vi "in loop button properties.vi"(0 "range settings":T1, 7 "range indicator refs":T2, 11 "error in (no error)":errorcluster) -> (15 "error out":errorcluster)   [LabVIEW 2014]
doc: "This subvi manages the boolean indicator properties inside the main temperature controller loop.\n\nPaul K Dixon\nPhysics 350\nPaul K Dixon"
uses:
  typedefs/status indicator.ctl
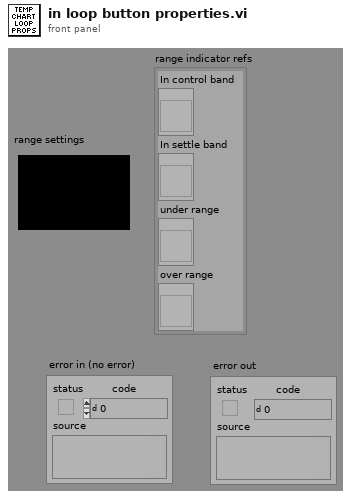
[diagram p1: front panel]
types:
  T1 = typedef "status indicator.ctl" = cluster{"In control band":bool, "In settle band":bool, "under range":bool, "over range":bool}
  T2 = cluster{"In control band":refnum<vi>, "In settle band":refnum<vi>, "under range":refnum<vi>, "over range":refnum<vi>}
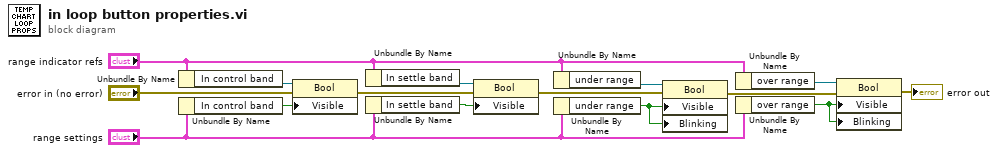
[diagram p0: block diagram]
diagram:
  n1 = Unbundle By Name("range indicator refs") -> ("In control band"=w15:refnum<vi>)
  n2 = Unbundle By Name("range settings") -> ("In control band"=w5:bool)
  n3 = property class="Bool"(reference=w15, error in="error in (no error)", "Visible"=w5) -> (error out=w12:errorcluster)  [unwired: 1 out]
  n4 = Unbundle By Name("range indicator refs") -> ("In settle band"=w13:refnum<vi>)
  n5 = Unbundle By Name("range settings") -> ("In settle band"=w3:bool)
  n6 = property class="Bool"(reference=w13, error in=w12, "Visible"=w3) -> (error out=w11:errorcluster)  [unwired: 1 out]
  n7 = Unbundle By Name("range indicator refs") -> ("under range"=w10:refnum<vi>)
  n8 = Unbundle By Name("range settings") -> ("under range"=w2:bool)
  n9 = property class="Bool"(reference=w10, error in=w11, "Visible"=w2, "Blinking"=w2) -> (error out=w7:errorcluster)  [unwired: 1 out]
  n10 = Unbundle By Name("range indicator refs") -> ("over range"=w9:refnum<vi>)
  n11 = Unbundle By Name("range settings") -> ("over range"=w1:bool)
  n12 = property class="Bool"(reference=w9, error in=w7, "Visible"=w1, "Blinking"=w1) -> (error out=→"error out":errorcluster)  [unwired: 1 out]
